vi "Do Clear Selection List.vi"(8 "error in (no error)":errorcluster, 10 "input cluster":T1, 11 "Data Cluster in":T2) -> (0 "error out":errorcluster, 3 "Data Cluster out":T2)   [LabVIEW 2025, in "Scripting Server.lvlib"]
uses:
  Scripting Server.lvlib
  Module Data--cluster.ctl
  clear_selection_list (Reply Payload)--cluster.ctl
  clear_selection_list Argument--cluster.ctl
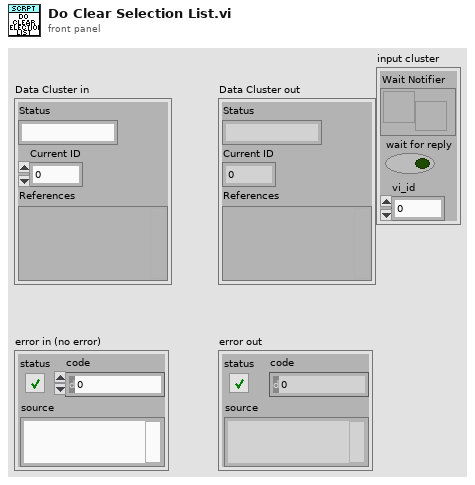
[diagram p1: front panel]
types:
  T1 = typedef "Scripting Server.lvlib/clear_selection_list Argument--cluster.ctl" = cluster{"Wait Notifier":refnum<notifier>, "wait for reply":bool, "vi_id":i32}
  T2 = typedef "Scripting Server.lvlib/Module Data--cluster.ctl" = cluster{"Status":string, "Current ID":i32, "References":variant}
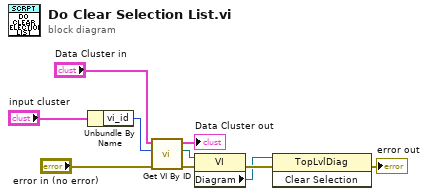
[diagram p0: block diagram]
diagram:
  n1 = Unbundle By Name("input cluster") -> ("vi_id"=w5:i32)
  n2 = call "Get VI By ID.vi"("error in (no error)"="error in (no error)", "ID"=w5, "Data Cluster in"="Data Cluster in") -> ("error out"=w8:errorcluster, "VI Reference"=w3:refnum<vi>, "Data Cluster out"=→"Data Cluster out":T2)  [unwired: 6 in]
  n3 = property class="VI"(reference=w3, error in=w8) -> (error out=w4:errorcluster, "Diagram"=w1:refnum<vi>)  [unwired: 1 out]
  n4 = invoke class="TopLvlDiag" method="Clear Selection"(reference=w1, error in=w4) -> (error out=→"error out":errorcluster)  [unwired: 1 in, 2 out]
